vi "NPL Joerger find max values.vi"(11 "Input":ext[][](array[numeric])) -> (1 "Electrons Min Value":ext[](array[numeric]), 3 "Ions Max Value":ext[](array[numeric]))   [LabVIEW 2013]
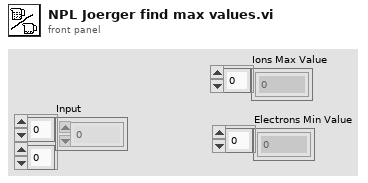
[diagram p1: front panel]
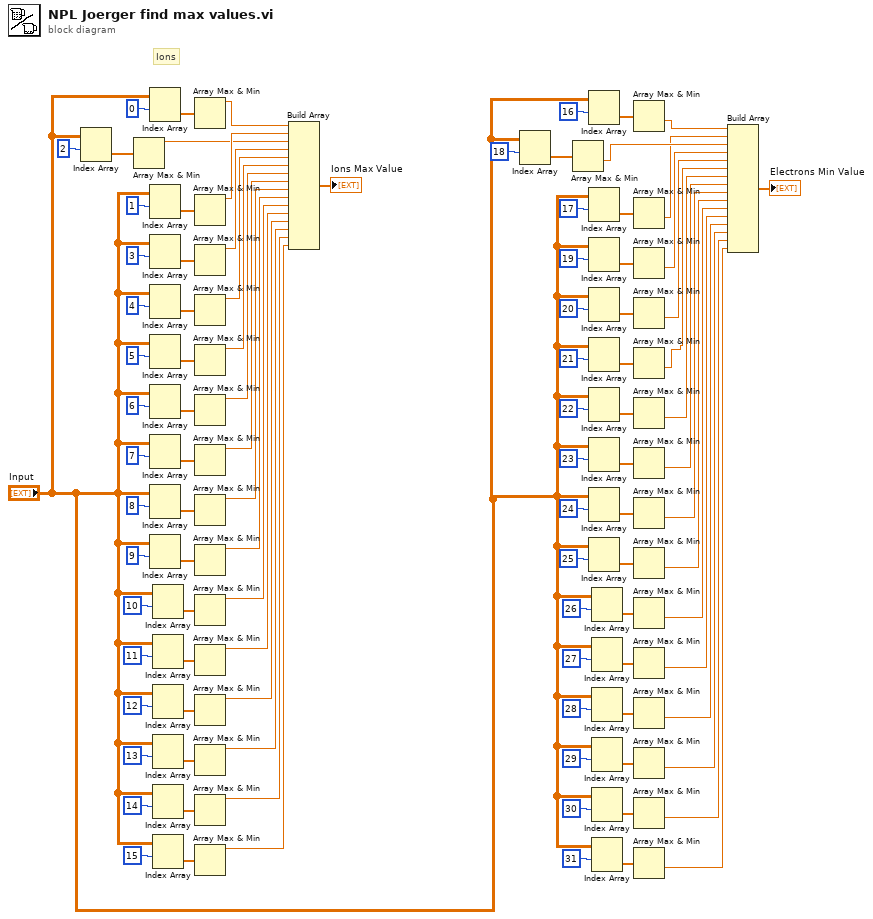
[diagram p0: block diagram]
diagram:
  # "Ions"
  n1 = Index Array(array="Input", index (row)=2) -> (element=w81:ext[])  [unwired: 1 in]
  n2 = Array Max & Min(array=w81) -> (max value=w65:ext)  [unwired: 3 out]
  n3 = Index Array(array="Input", index (row)=0) -> (element=w83:ext[])  [unwired: 1 in]
  n4 = Index Array(array="Input", index (row)=1) -> (element=w82:ext[])  [unwired: 1 in]
  n5 = Index Array(array="Input", index (row)=3) -> (element=w80:ext[])  [unwired: 1 in]
  n6 = Index Array(array="Input", index (row)=4) -> (element=w79:ext[])  [unwired: 1 in]
  n7 = Index Array(array="Input", index (row)=5) -> (element=w78:ext[])  [unwired: 1 in]
  n8 = Index Array(array="Input", index (row)=6) -> (element=w77:ext[])  [unwired: 1 in]
  n9 = Index Array(array="Input", index (row)=7) -> (element=w76:ext[])  [unwired: 1 in]
  n10 = Index Array(array="Input", index (row)=8) -> (element=w75:ext[])  [unwired: 1 in]
  n11 = Index Array(array="Input", index (row)=9) -> (element=w74:ext[])  [unwired: 1 in]
  n12 = Index Array(array="Input", index (row)=10) -> (element=w73:ext[])  [unwired: 1 in]
  n13 = Index Array(array="Input", index (row)=11) -> (element=w72:ext[])  [unwired: 1 in]
  n14 = Index Array(array="Input", index (row)=12) -> (element=w71:ext[])  [unwired: 1 in]
  n15 = Index Array(array="Input", index (row)=13) -> (element=w70:ext[])  [unwired: 1 in]
  n16 = Index Array(array="Input", index (row)=14) -> (element=w69:ext[])  [unwired: 1 in]
  n17 = Index Array(array="Input", index (row)=15) -> (element=w68:ext[])  [unwired: 1 in]
  n18 = Array Max & Min(array=w83) -> (max value=w67:ext)  [unwired: 3 out]
  n19 = Array Max & Min(array=w82) -> (max value=w66:ext)  [unwired: 3 out]
  n20 = Array Max & Min(array=w80) -> (max value=w64:ext)  [unwired: 3 out]
  n21 = Array Max & Min(array=w79) -> (max value=w63:ext)  [unwired: 3 out]
  n22 = Array Max & Min(array=w78) -> (max value=w62:ext)  [unwired: 3 out]
  n23 = Array Max & Min(array=w77) -> (max value=w61:ext)  [unwired: 3 out]
  n24 = Array Max & Min(array=w76) -> (max value=w60:ext)  [unwired: 3 out]
  n25 = Array Max & Min(array=w75) -> (max value=w59:ext)  [unwired: 3 out]
  n26 = Array Max & Min(array=w74) -> (max value=w58:ext)  [unwired: 3 out]
  n27 = Array Max & Min(array=w73) -> (max value=w57:ext)  [unwired: 3 out]
  n28 = Array Max & Min(array=w72) -> (max value=w56:ext)  [unwired: 3 out]
  n29 = Array Max & Min(array=w71) -> (max value=w55:ext)  [unwired: 3 out]
  n30 = Array Max & Min(array=w70) -> (max value=w54:ext)  [unwired: 3 out]
  n31 = Array Max & Min(array=w69) -> (max value=w53:ext)  [unwired: 3 out]
  n32 = Array Max & Min(array=w68) -> (max value=w52:ext)  [unwired: 3 out]
  n33 = Build Array(w67, w66, w65, w64, w63, w62, w61, w60, w59, w58, w57, w56, w55, w54, w53, w52) -> (→"Ions Max Value":ext[])
  n34 = Index Array(array="Input", index (row)=18) -> (element=w36:ext[])  [unwired: 1 in]
  n35 = Array Max & Min(array=w36) -> (min value=w15:ext)  [unwired: 3 out]
  n36 = Index Array(array="Input", index (row)=16) -> (element=w34:ext[])  [unwired: 1 in]
  n37 = Index Array(array="Input", index (row)=17) -> (element=w35:ext[])  [unwired: 1 in]
  n38 = Index Array(array="Input", index (row)=19) -> (element=w37:ext[])  [unwired: 1 in]
  n39 = Index Array(array="Input", index (row)=20) -> (element=w38:ext[])  [unwired: 1 in]
  n40 = Index Array(array="Input", index (row)=21) -> (element=w39:ext[])  [unwired: 1 in]
  n41 = Index Array(array="Input", index (row)=22) -> (element=w40:ext[])  [unwired: 1 in]
  n42 = Index Array(array="Input", index (row)=23) -> (element=w41:ext[])  [unwired: 1 in]
  n43 = Index Array(array="Input", index (row)=24) -> (element=w42:ext[])  [unwired: 1 in]
  n44 = Index Array(array="Input", index (row)=25) -> (element=w43:ext[])  [unwired: 1 in]
  n45 = Index Array(array="Input", index (row)=26) -> (element=w44:ext[])  [unwired: 1 in]
  n46 = Index Array(array="Input", index (row)=27) -> (element=w45:ext[])  [unwired: 1 in]
  n47 = Index Array(array="Input", index (row)=28) -> (element=w46:ext[])  [unwired: 1 in]
  n48 = Index Array(array="Input", index (row)=29) -> (element=w47:ext[])  [unwired: 1 in]
  n49 = Index Array(array="Input", index (row)=30) -> (element=w48:ext[])  [unwired: 1 in]
  n50 = Index Array(array="Input", index (row)=31) -> (element=w49:ext[])  [unwired: 1 in]
  n51 = Array Max & Min(array=w34) -> (min value=w16:ext)  [unwired: 3 out]
  n52 = Array Max & Min(array=w35) -> (min value=w14:ext)  [unwired: 3 out]
  n53 = Array Max & Min(array=w37) -> (min value=w13:ext)  [unwired: 3 out]
  n54 = Array Max & Min(array=w38) -> (min value=w12:ext)  [unwired: 3 out]
  n55 = Array Max & Min(array=w39) -> (min value=w11:ext)  [unwired: 3 out]
  n56 = Array Max & Min(array=w40) -> (min value=w10:ext)  [unwired: 3 out]
  n57 = Array Max & Min(array=w41) -> (min value=w9:ext)  [unwired: 3 out]
  n58 = Array Max & Min(array=w42) -> (min value=w8:ext)  [unwired: 3 out]
  n59 = Array Max & Min(array=w43) -> (min value=w7:ext)  [unwired: 3 out]
  n60 = Array Max & Min(array=w44) -> (min value=w6:ext)  [unwired: 3 out]
  n61 = Array Max & Min(array=w45) -> (min value=w5:ext)  [unwired: 3 out]
  n62 = Array Max & Min(array=w46) -> (min value=w4:ext)  [unwired: 3 out]
  n63 = Array Max & Min(array=w47) -> (min value=w3:ext)  [unwired: 3 out]
  n64 = Array Max & Min(array=w48) -> (min value=w2:ext)  [unwired: 3 out]
  n65 = Array Max & Min(array=w49) -> (min value=w1:ext)  [unwired: 3 out]
  n66 = Build Array(w16, w14, w15, w13, w12, w11, w10, w9, w8, w7, w6, w5, w4, w3, w2, w1) -> (→"Electrons Min Value":ext[])
